vi "Connect to Artifactory.vi"(5 "Artifactory in":refnum<class "Artifactory.lvclass">, 6 "Authorization":T2={"auth-type"=enum."API Key", "username"="", "api-key"=""}, 8 "error in (no error)":errorcluster, 9 "repository path":string, 10 "server-uri":string, 11 "Local Repository":path) -> (0 "error out":errorcluster, 2 "Public Events":T1, 3 "Artifactory out":refnum<class "Artifactory.lvclass">)   [LabVIEW 2021, in "Artifactory.lvclass"]
uses:
  Artifactory.lvclass
  Authorization -- cluster.ctl
  auth-type -- enum.ctl
  Public Events -- cluster.ctl
  Repository Event -- cluster.ctl
  Actions -- enum.ctl
  <vilib>/addons/_JKI.lib/REST Client/classes/REST Client/HTTP Header.ctl
  Artifactory.lvclass/Artifactory.ctl
  <vilib>/LabVIEW Open Source Project/OpenSerializer.Base64/Base64_CharSet.vi
  <vilib>/addons/_JKI.lib/REST Client/classes/REST Client/REST Client.lvclass
  <vilib>/LabVIEW Open Source Project/OpenSerializer.Base64/Serializer.Base64.lvclass
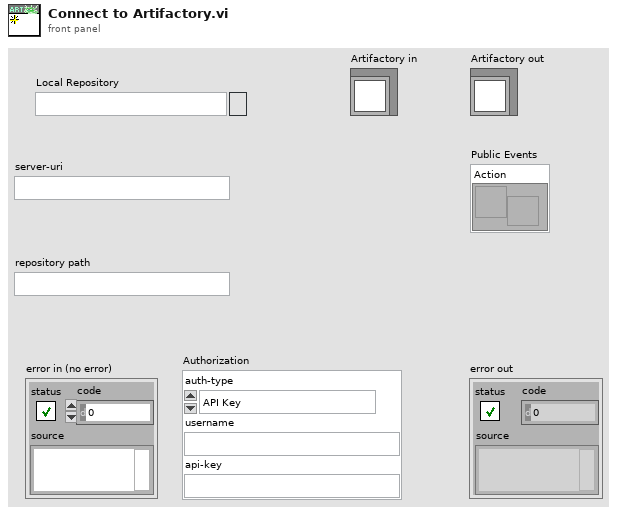
[diagram p1: front panel]
types:
  T1 = typedef "Artifactory.lvclass/Public Events -- cluster.ctl" = cluster{"Action":refnum<user-event>}
  T2 = typedef "Artifactory.lvclass/Authorization -- cluster.ctl" = cluster{"auth-type":T3, "username":string, "api-key":string}
  T3 = typedef "Artifactory.lvclass/auth-type -- enum.ctl" = enum16{"Username + Password", "Username + API Key", "API Key", "Access token"}
  T4 = typedef "REST Client.lvlib/REST Client.lvclass/HTTP Header.ctl" = cluster{"header":string, "value":string}
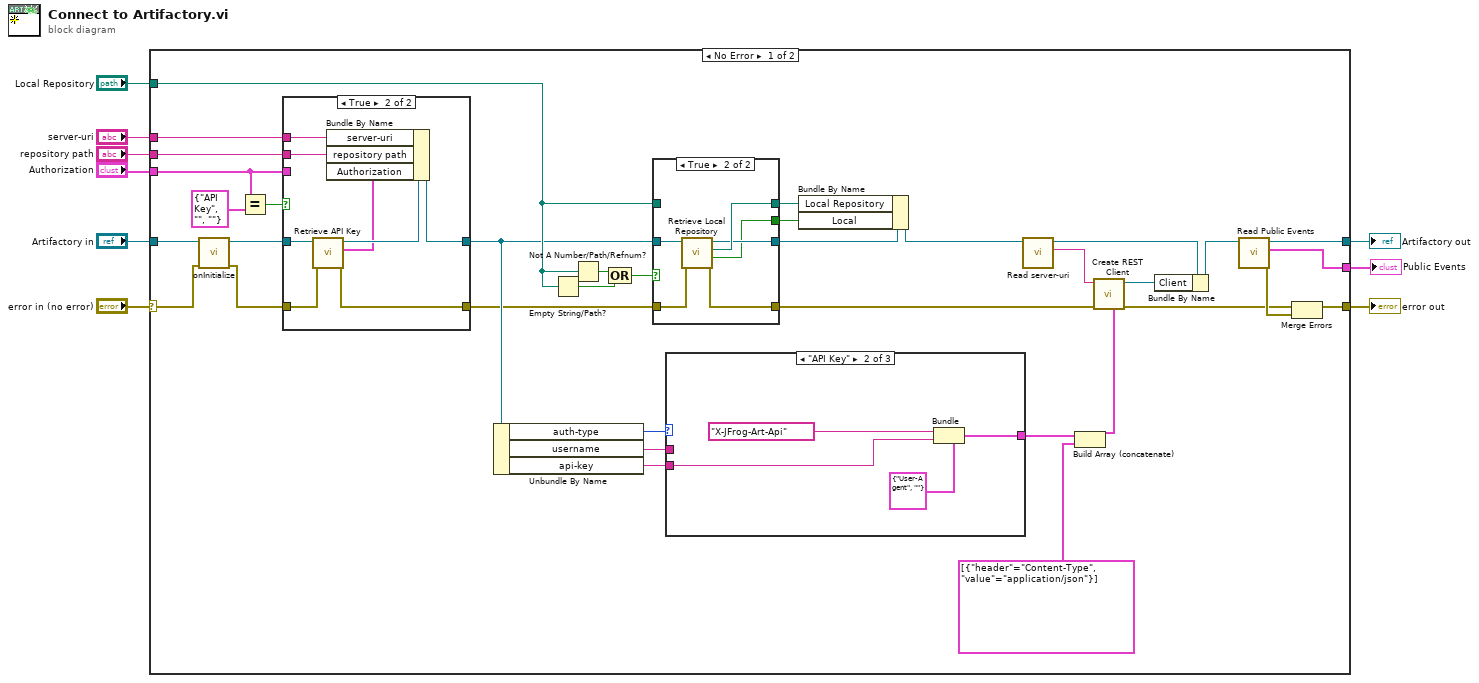
[diagram p0: block diagram]
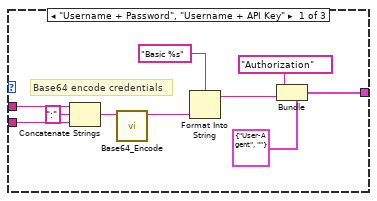
[diagram p2: hidden frame]
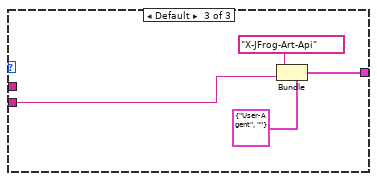
[diagram p3: hidden frame]
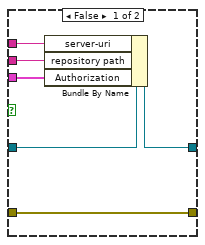
[diagram p5: hidden frame]
diagram:
  n1 = case shown="No Error" "error in (no error)" {
    selector: "error in (no error)" -> [w17 w87]
    tunnel: [w10 w87] -> w8
    tunnel: [w13 w86] -> w6
    tunnel: "Artifactory in" -> [w18 w86]
    tunnel: "Local Repository" -> [w26 _]
    tunnel: "server-uri" -> [w36 _]
    tunnel: "repository path" -> [w35 _]
    tunnel: "Authorization" -> [w34 _]
    tunnel: [w15 _] -> w1
    frame No Error {
      n2 = call-dynamic "onInitialize.vi"("error in (no error)"=w17, "Artifactory in"=w18) -> ("error out"=w16:errorcluster, "Artifactory out"=w19:refnum<class "Artifactory.lvclass">)  [unwired: 8 in]
      n3 = Equal?(x=w34, y=T2 {"auth-type"=enum."API Key", "username"="", "api-key"=""} ("Basic Authorization")) -> (x = y?=w32:bool)
      n4 = case shown="True" w32 {
        tunnel: [w77 w85] -> w24
        tunnel: w36 -> [w76 w84]
        tunnel: w35 -> [w75 w83]
        tunnel: w19 -> [w74 w79]
        tunnel: w34 -> [w73 _]
        tunnel: [w72 w82] -> w23
        tunnel: w16 -> [w72 w81]
        frame False {
          n5 = Bundle By Name(cluster=w74, "server-uri"=w76, "repository path"=w75, "Authorization"=w73) -> (w77:refnum<class "Artifactory.lvclass">)
        }
        frame True {
          n6 = call-dynamic "Retrieve API Key.vi"("error in"=w81, "Artifactory"=w79) -> ("error out"=w82:errorcluster, "Authorization"=w78:T2, "Artifactory out"=w80:refnum<class "Artifactory.lvclass">)  [unwired: 6 in, 1 out]
          n7 = Bundle By Name(cluster=w80, "server-uri"=w84, "repository path"=w83, "Authorization"=w78) -> (w85:refnum<class "Artifactory.lvclass">)
        }
      }
      n8 = Unbundle By Name(w24) -> ("auth-type"=w21:T3, "username"=w41:string, "api-key"=w40:string)
      n9 = Empty String/Path?(string/path=w26) -> (empty?=w29:bool)
      n10 = Not A Number/Path/Refnum?(number/path/refnum=w26) -> (NaN/Path/Refnum?=w30:bool)
      n11 = Compound Arithmetic op=OR(w30, w29) -> (w28:bool)
      n12 = case shown="True" w28 {
        tunnel: [w65 w71] -> w27
        tunnel: w26 -> [w65 _]
        tunnel: [w64 w69] -> w25
        tunnel: w24 -> [w64 w70]
        tunnel: w23 -> [w63 w68]
        tunnel: [w63 w67] -> w22
        tunnel: [_ w66] -> w20
        frame False {
        }
        frame True {
          n13 = call-dynamic "Retrieve Local Repository.vi"("error in"=w68, "Artifactory"=w70) -> ("error out"=w67:errorcluster, "found"=w66:bool, "Local Repository"=w71:path, "Artifactory out"=w69:refnum<class "Artifactory.lvclass">)  [unwired: 6 in]
        }
      }
      n14 = case shown="\"API Key\"" w21 {
        tunnel: [w54 w58 w62] -> w43
        tunnel: w41 -> [w48 _ _]
        tunnel: w40 -> [w47 w55 w59]
        frame "Username + Password", "Username + API Key" {
          # "Base64 encode credentials"
          n15 = Concatenate Strings(w48, ":" ("string"), w47) -> (w46:string)
          n16 = call <vilib>:"Base64_Encode.vi"("String"=w46) -> ("Encoded String"=w49:string)  [unwired: 9 in, 1 out]
          n17 = Format Into String(format string="Basic %s" ("value"), w49) -> (resulting string=w50:string)  [unwired: 2 in, 1 out]
          n18 = Bundle(cluster=T4 {"header"="User-Agent", "value"=""} ("Header"), "header"="Authorization", "value"=w50) -> (w54:T4)
        }
        frame "API Key" {
          n19 = Bundle(cluster=T4 {"header"="User-Agent", "value"=""} ("Header"), "header"="X-JFrog-Art-Api", "value"=w55) -> (w58:T4)
        }
        frame Default {
          n20 = Bundle(cluster=T4 {"header"="User-Agent", "value"=""} ("Header"), "header"="X-JFrog-Art-Api", "value"=w59) -> (w62:T4)
        }
      }
      n21 = Bundle By Name(cluster=w25, "Local Repository"=w27, "Local"=w20) -> (w31:refnum<class "Artifactory.lvclass">)
      n22 = call "Read server-uri.vi"("Artifactory in"=w31) -> ("server-uri"=w39:string, "Artifactory out"=w38:refnum<class "Artifactory.lvclass">)  [unwired: 9 in]
      n23 = Build Array (concatenate)(w43, T4[] [{"header"="Content-Type", "value"="application/json"}] ("Default Headers ([JSON])")) -> (w37:T4[])
      n24 = call <vilib>:"Create REST Client.vi"("Default Headers ([JSON])"=w37, "error in (no error)"=w22, "Base URL"=w39) -> ("error out"=w11:errorcluster, "REST Client out"=w44:refnum<class "REST Client.lvclass">)  [unwired: 7 in]
      n25 = Bundle By Name(cluster=w38, "Client"=w44) -> (w14:refnum<class "Artifactory.lvclass">)
      n26 = call-dynamic "Read Public Events.vi"("Artifactory in"=w14) -> ("error out"=w12:errorcluster, "Public Events"=w15:T1, "Artifactory out"=w13:refnum<class "Artifactory.lvclass">)  [unwired: 8 in]
      n27 = Merge Errors(w11, w12) -> (w10:errorcluster)
    }
    frame Error {
    }
  }
  "error out" <- w8
  "Artifactory out" <- w6
  "Public Events" <- w1
